vi "Do.vi"(8 "error in (no error)":errorcluster, 10 "Actor in":refnum<class "Actor.lvclass">, 11 "Status Update Msg":refnum<class "Status Update Msg.lvclass">) -> (0 "error out":errorcluster, 2 "Actor out":refnum<class "Actor.lvclass">)   [LabVIEW 2020, in "Server.lvlib" / "Status Update Msg.lvclass"]
doc: "This VI delivers the message to the actor by calling the appropriate method(s) on the actor."
uses:
  Status Update Msg.lvclass
  C:/Users/huipeng8/Desktop/Chat-Window-Tutorial-Series/Video 11 - Actor Sub-panels/Chat Window Model/Chat Window Model Messages/Status Updated Msg/Status Updated Msg.lvclass
  <vilib>/ActorFramework/Actor/Actor.lvclass
  Server/Server.lvclass
  C:/Program Files/National Instruments/LabVIEW 2020/vi.lib/ActorFramework/Actor/Actor.lvclass
  Chat Window Model/Chat Window Model Messages/Status Updated Msg/Status Updated Msg.lvclass/Status Updated Msg.ctl
  Chat Window Model/Chat Window Model Messages/Status Updated Msg/Status Updated Msg.lvclass
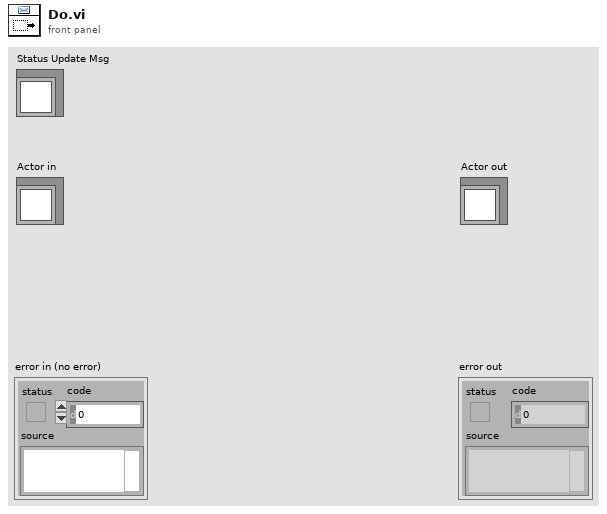
[diagram p1: front panel]
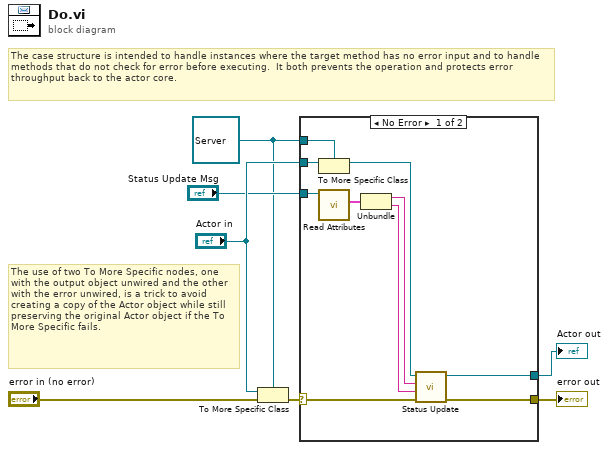
[diagram p0: block diagram]
diagram:
  w2 = refnum<class "Server.lvclass"> refnum ("Actor in")
  # "The use of two To More Specific nodes, one with the output object unwired and the other with the error unwired, is a trick to avoid creating a copy of the Actor object while still preserving the original Actor object if the To More Specific fails."
  # "The case structure is intended to handle instances where the target method has no error input and to handle methods that do not check for error before executing.  It both prevents the operation and protects error throughput back to the actor core."
  n1 = To More Specific Class(target class=w2, reference="Actor in", error in="error in (no error)") -> (error out=w1:errorcluster)  [unwired: 1 out]
  n2 = case shown="No Error" w1 {
    selector: w1 -> [w15 w19]
    tunnel: [w17 w19] -> w7
    tunnel: [w16 w18] -> w6
    tunnel: "Actor in" -> [w14 w18]
    tunnel: w2 -> [w13 _]
    tunnel: "Status Update Msg" -> [w10 _]
    frame No Error {
      n3 = To More Specific Class(target class=w13, reference=w14) -> (specific class reference=w12:refnum<class "Server.lvclass">)  [unwired: 1 in, 1 out]
      n4 = call "Read Attributes.vi"("Status Updated Msg"=w10) -> ("Payload"=w11:cluster{"Name":string, "Status":string})  [unwired: 10 in]
      n5 = Unbundle(w11) -> ("Name"=w9:string, "Status"=w8:string)
      n6 = call "Status Update.vi"("error in (no error)"=w15, "Status"=w8, "Name"=w9, "Server in"=w12) -> ("error out"=w17:errorcluster, "Server out"=w16:refnum<class "Server.lvclass">)  [unwired: 6 in]
    }
    frame Error {
      # "If type check fails, pass the original object out again."
    }
  }
  "error out" <- w7
  "Actor out" <- w6
